vi "Initialize From Settings.vi"(8 "error in":errorcluster, 10 "settings":cluster{"key":string, "value":string}[](array[cluster]), 11 "RDMA Rx Transfer Configuration in":refnum<class "RDMA Transfer Rx Configuration.lvclass">) -> (0 "error out":errorcluster, 3 "RDMA Rx Transfer Configuration out":refnum<class "RDMA Transfer Rx Configuration.lvclass">)   [LabVIEW 2020, in "RDMA.lvlib" / "RDMA Transfer Rx Configuration.lvclass"]
uses:
  RDMA Transfer Rx Configuration.lvclass
  Rx Transfer Settings.ctl
  RDMA Transfer Rx Configuration.lvclass/RDMA Transfer Rx Configuration.ctl
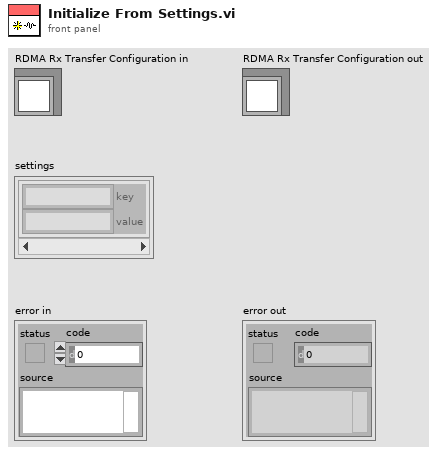
[diagram p1: front panel]
types:
  T1 = typedef "RDMA.lvlib/RDMA Transfer Rx Configuration.lvclass/Rx Transfer Settings.ctl" = cluster{"local address":u32, "local port":u16, "decimation":u16}
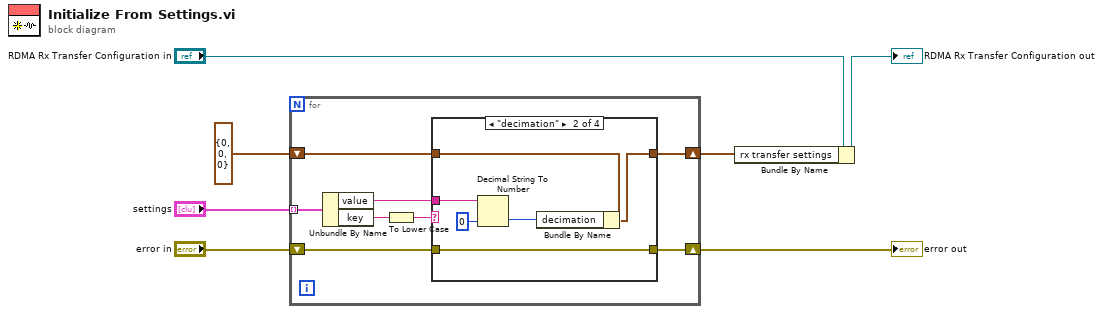
[diagram p0: block diagram]
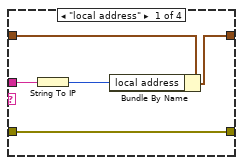
[diagram p2: hidden frame]
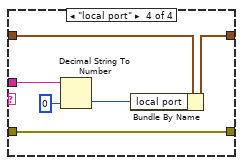
[diagram p4: hidden frame]
diagram:
  n1 = for {
    shift-right: [w10] -> w1
    shift-left: "error in" -> [w14]
    shift-right: [w12] -> w5
    shift-left: T1 {"local address"=0, "local port"=0, "decimation"=0} ("rx transfer settings") -> [w13]
    tunnel: "settings" -> [w15] mode=indexing
    n2 = Unbundle By Name(w15) -> ("value"=w9:string, "key"=w8:string)
    n3 = To Lower Case(string=w8) -> (all lower case string=w11:string)
    n4 = case shown="\"decimation\"" w11 {
      tunnel: w14 -> [w18 w24 w27 w32]
      tunnel: w9 -> [w17 w22 _ w31]
      tunnel: w13 -> [w20 w26 w28 w34]
      tunnel: [w19 w25 w28 w33] -> w12
      tunnel: [w18 w24 w27 w32] -> w10
      frame "local address" {
        n5 = String To IP(1:w17) -> (0:w16:u32)
        n6 = Bundle By Name(cluster=w20, "local address"=w16) -> (w19:T1)
      }
      frame "decimation" {
        n7 = Decimal String To Number(string=w22, default (0L)=u16 0 ("default (0 I32)")) -> (number=w21:u16)  [unwired: 1 in, 1 out]
        n8 = Bundle By Name(cluster=w26, "decimation"=w21) -> (w25:T1)
      }
      frame Default {
        # "Unknown Setting:\nmay need to throw\nan error here"
      }
      frame "local port" {
        n9 = Decimal String To Number(string=w31, default (0L)=u16 0 ("default (0 I32)")) -> (number=w30:u16)  [unwired: 1 in, 1 out]
        n10 = Bundle By Name(cluster=w34, "local port"=w30) -> (w33:T1)
      }
    }
  }
  "error out" <- w1
  n11 = Bundle By Name(cluster="RDMA Rx Transfer Configuration in", "rx transfer settings"=w5) -> (→"RDMA Rx Transfer Configuration out":refnum<class "RDMA Transfer Rx Configuration.lvclass">)
